vi "Setup Camera.vi"(9 "Image Settings":T4={"Image Size"=enum."160x120", "Frame Rate (fps)"=0.0, "White Balance"=enum."Fixed fluorescent 1", "Exposure"=enum."Auto", "Compression"=40, "Brightness"=76}, 11 "Camera RefNum":string="Camera") -> (0 "error out":errorcluster)   [LabVIEW 2012]
uses:
  <vilib>/Rock Robotics/WPI/Camera/WPI_CameraImageSize.ctl
  <vilib>/Rock Robotics/WPI/Camera/WPI_CameraWhite Balance Values.ctl
  <vilib>/Rock Robotics/WPI/Camera/WPI_CameraExposure Values.ctl
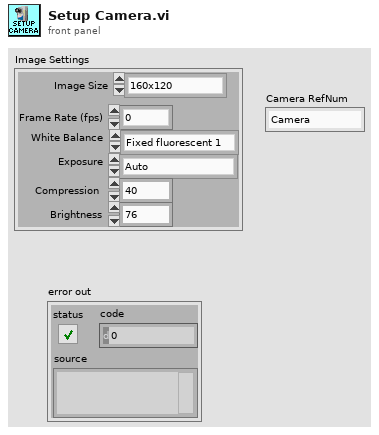
[diagram p1: front panel]
types:
  T1 = typedef "WPI_CameraImageSize.ctl" = enum16{"640x480", "320x240", "160x120"}
  T2 = typedef "WPI_CameraWhite Balance Values.ctl" = enum16{"Auto", "Fixed indoor", "Fixed outdoor 1", "Fixed outdoor 2", "Fixed fluorescent 1", "Fixed fluorescent 2", "Hold current"}
  T3 = typedef "WPI_CameraExposure Values.ctl" = enum16{"Auto", "Flicker-free 50 Hz", "Flicker-free 60 Hz", "Hold current"}
  T4 = cluster{"Image Size":T1, "Frame Rate (fps)":dbl, "White Balance":T2, "Exposure":T3, "Compression":i32, "Brightness":i32}
  T5 = typedef "WPI_CameraDevRef.ctl" = cluster{"Camera Address":string, "CameraStatus":errorcluster, "Acquire Image Notifier":refnum<notifier>}
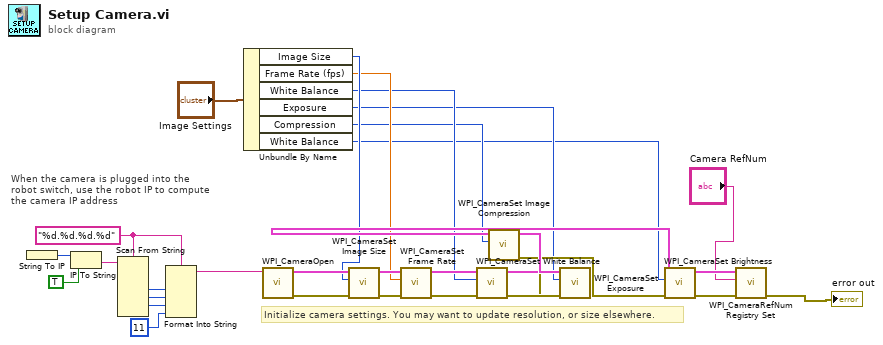
[diagram p0: block diagram]
diagram:
  w11 = "%d.%d.%d.%d" ("format string")
  # "When the camera is plugged into the\nrobot switch, use the robot IP to compute\nthe camera IP address"
  # "Initialize camera settings. You may want to update resolution, or size elsewhere."
  n1 = String To IP() -> (0:w18:u32)  [unwired: 1 in]
  n2 = IP To String(1:TRUE ("dot notation? (F)"), 2:w18) -> (0:w16:string)
  n3 = Scan From String(format string=w11, input string=w16) -> (output 1=w15:i32, output 2=w14:i32, output 3=w13:i32)  [unwired: 7 in, 3 out]
  n4 = Format Into String(format string=w11, w15, w14, w13, 11 ("Compression")) -> (resulting string=w10:string)  [unwired: 2 in, 1 out]
  n5 = Unbundle By Name("Image Settings") -> ("Image Size"=w6:T1, "Frame Rate (fps)"=w5:dbl, "White Balance"=w4:T2, "Exposure"=w3:T3, "Compression"=w2:i32, "White Balance"=w1:T2)
  n6 = call <vilib>:"WPI_CameraOpen.vi"("Camera Address"=w10) -> ("error out"=w26:errorcluster, "CameraDevRef"=w27:T5)  [unwired: 1 in, 8 out]
  n7 = call <vilib>:"WPI_CameraSet Image Size.vi"("error in (no error)"=w26, "Image Size"=w6, "CameraDevRef"=w27) -> ("error out"=w25:errorcluster, "CameraDevRef Out"=w28:T5)  [unwired: 7 out]
  n8 = call <vilib>:"WPI_CameraSet Frame Rate.vi"("error in (no error)"=w25, "Frame Rate (fps)"=w5, "CameraDevRef"=w28) -> ("error out"=w24:errorcluster, "CameraDevRef Out"=w30:T5)  [unwired: 7 out]
  n9 = call <vilib>:"WPI_CameraSet White Balance.vi"("error in (no error)"=w24, "White Balance"=w4, "CameraDevRef"=w30) -> ("error out"=w23:errorcluster, "CameraDevRef Out"=w29:T5)  [unwired: 7 out]
  n10 = call <vilib>:"WPI_CameraSet Exposure.vi"("error in (no error)"=w23, "Exposure"=w3, "CameraDevRef"=w29) -> ("error out"=w22:errorcluster, "CameraDevRef Out"=w32:T5)  [unwired: 7 out]
  n11 = call <vilib>:"WPI_CameraSet Image Compression.vi"("error in (no error)"=w22, "Compression"=w2, "CameraDevRef"=w32) -> ("error out"=w21:errorcluster, "CameraDevRef Out"=w31:T5)  [unwired: 7 out]
  n12 = call <vilib>:"WPI_CameraSet Brightness.vi"("error in (no error)"=w21, "Brightness"=w1, "CameraDevRef"=w31) -> ("error out"=w19:errorcluster, "CameraDevRef Out"=w20:T5)  [unwired: 7 out]
  n13 = call <vilib>:"WPI_CameraRefNum Registry Set.vi"("error in (no error)"=w19, "refnum name"="Camera RefNum", "CameraDevRef"=w20) -> ("error out"=→"error out":errorcluster)  [unwired: 8 out]
